vi "sub_CMC Match.vi"(8 "error in (no error)":errorcluster caption="에러 입력(에러 없음)", 10 "DATA IN":string[][](array[string]), 11 "CMC IN":string[][](array[string])) -> (0 "error out":errorcluster caption="에러 출력", 2 "에러?":bool, 3 "CMC Out":string[][](array[string]))   [LabVIEW 2020]
panel:
  out "배열":bool[](array[boolean])
  # "0, DSEQ\n1, CLSMAN\n2, CLSMAN_EXT\n3, FUNC\n4, FUNC_EXT\n5, FUNC_CON\n6, C1_LOW\n7, C1_LUNIT\n8, C1_LCON\n9, C1_HIGH\n10, C1_HUNIT\n11, C1_HCON\n12, RANGE_LOW\n13, RANGE_LUNIT\n14, RANGE_LDIV\n15, RANGE_HIGH\n16, RANGE_HUNIT\n17, RANGE_HDIV\n18, CMC1_VAL\n19, CMC2_VAL\n20, CMC_UNIT"
  # "0, CLSMAN_EXT\n1, FUNC\n2, FUNC_EXT\n3, FUNC_CON\n4, C1_VAL\n5, C1_UNIT\n6, RANGE_VAL\n7, RANGE_UNIT"
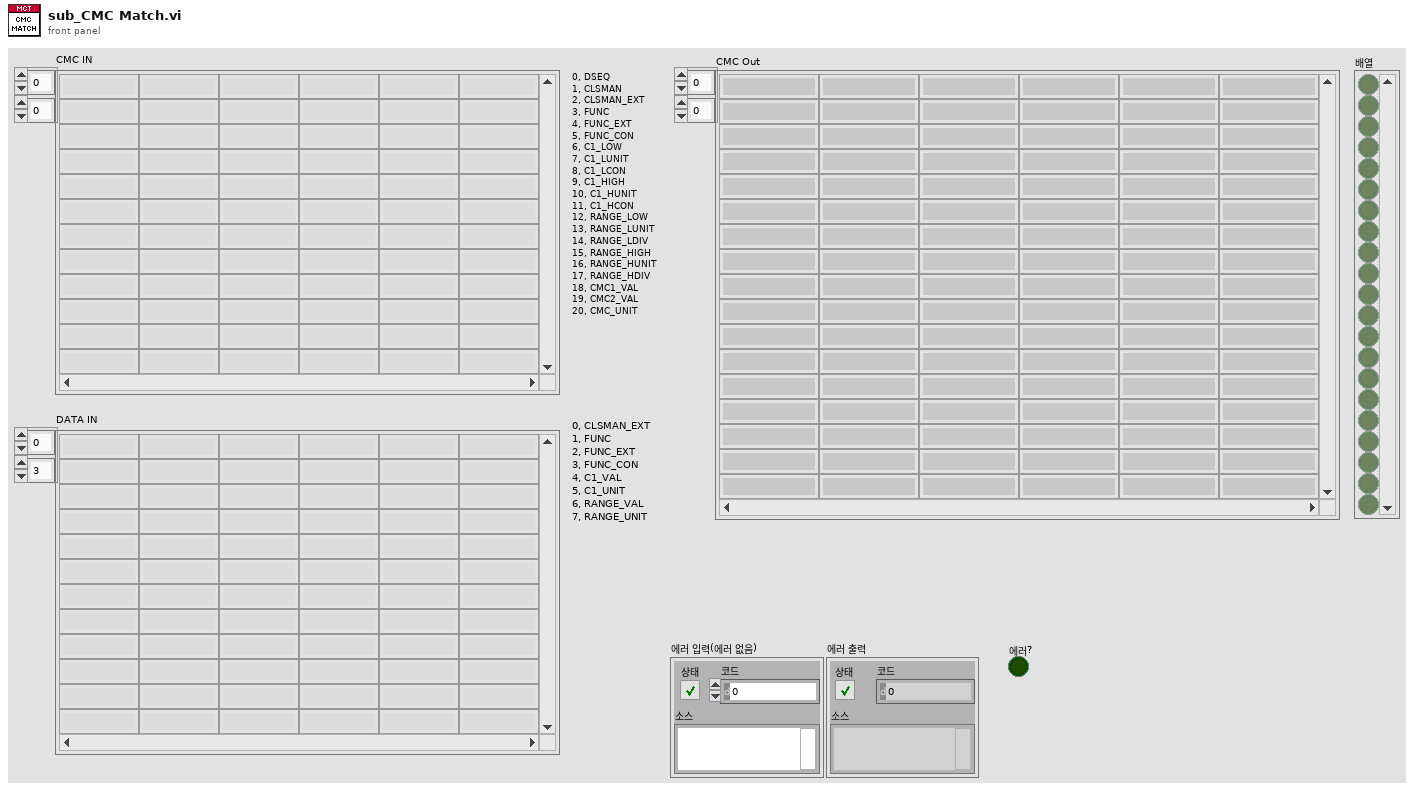
[diagram p1: front panel]
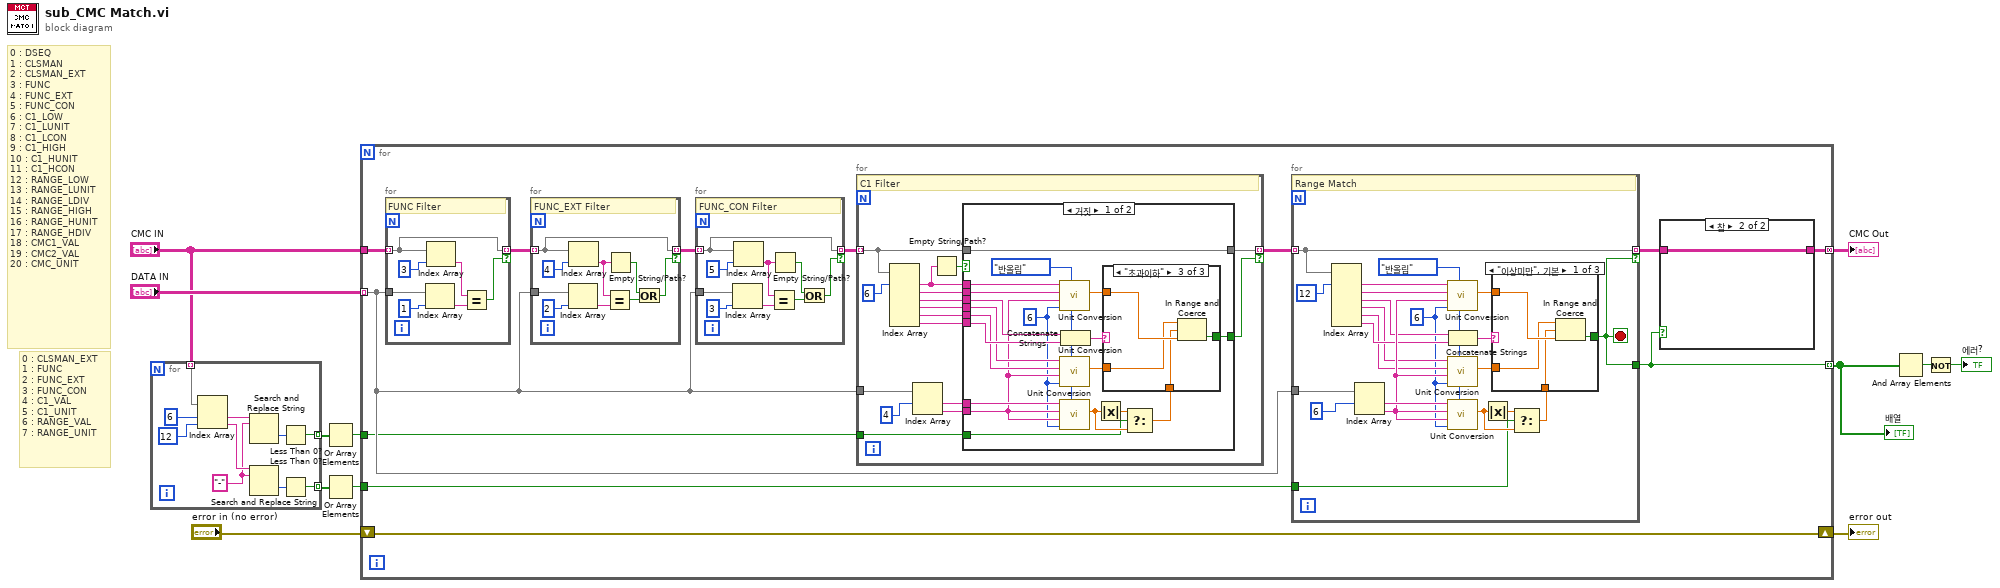
[diagram p0: block diagram]
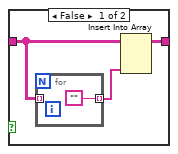
[diagram p2: hidden frame]
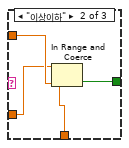
[diagram p3: hidden frame]
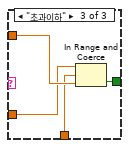
[diagram p4: hidden frame]
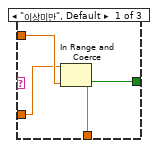
[diagram p5: hidden frame]
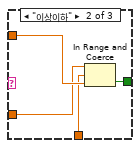
[diagram p6: hidden frame]
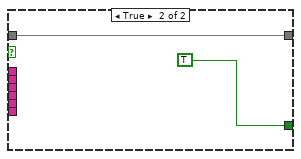
[diagram p7: hidden frame]
diagram:
  # "0 : CLSMAN_EXT\n1 : FUNC\n2 : FUNC_EXT\n3 : FUNC_CON\n4 : C1_VAL\n5 : C1_UNIT\n6 : RANGE_VAL\n7 : RANGE_UNIT"
  # "0 : DSEQ\n1 : CLSMAN\n2 : CLSMAN_EXT\n3 : FUNC\n4 : FUNC_EXT\n5 : FUNC_CON\n6 : C1_LOW\n7 : C1_LUNIT\n8 : C1_LCON\n9 : C1_HIGH\n10 : C1_HUNIT\n11 : C1_HCON\n12 : RANGE_LOW\n13 : RANGE_LUNIT\n14 : RANGE_LDIV\n15 : RANGE_HIGH\n16 : RANGE_HUNIT\n17 : RANGE_HDIV\n18 : CMC1_VAL\n19 : CMC2_VAL\n20 : CMC_UNIT"
  n1 = for {
    tunnel: "CMC IN" -> [w22] mode=indexing
    tunnel: [w18] -> w6 mode=indexing
    tunnel: [w13] -> w5 mode=indexing
    w15 = "-" ("검색 문자열")
    n2 = Index Array(array=w22, index #1=6 ("비활성화된 인덱스 (열)"), index #2=12 ("비활성화된 인덱스 (열)")) -> (element #1=w16:string, element #2=w20:string)
    n3 = Search and Replace String(input string=w16, search string=w15) -> (offset past replacement=w14:i32)  [unwired: 6 in, 3 out]
    n4 = Search and Replace String(input string=w20, search string=w15) -> (offset past replacement=w19:i32)  [unwired: 6 in, 3 out]
    n5 = Less Than 0?(x=w14) -> (x < 0?=w13:bool)
    n6 = Less Than 0?(x=w19) -> (x < 0?=w18:bool)
  }
  n7 = Or Array Elements(Boolean array=w5) -> (logical OR=w2:bool)
  n8 = Or Array Elements(Boolean array=w6) -> (logical OR=w1:bool)
  n9 = for {
    tunnel: "DATA IN" -> [w25] mode=indexing
    tunnel: "CMC IN" -> [w34]
    tunnel: [w28] -> w12 mode=concatenating
    shift-right: [w31] -> w10
    shift-left: "error in (no error)" -> [w31]
    tunnel: [w30] -> w9 mode=indexing
    tunnel: w2 -> [w24]
    tunnel: w1 -> [w23]
    n10 = for {
      tunnel: w34 -> [w146] mode=indexing
      tunnel: w25 -> [w147]
      tunnel: [w146] -> w33 mode=indexing if=w145
      # "FUNC Filter"
      n11 = Index Array(array=w147, index=1 ("인덱스")) -> (element=w143:string)
      n12 = Index Array(array=w146, index=3 ("인덱스")) -> (element=w144:string)
      n13 = Equal?(x=w144, y=w143) -> (x = y?=w145:bool)
    }
    n14 = for {
      tunnel: w33 -> [w139] mode=indexing
      tunnel: w25 -> [w140]
      tunnel: [w139] -> w27 mode=indexing if=w132
      # "FUNC_EXT Filter"
      n15 = Index Array(array=w140, index=2 ("인덱스")) -> (element=w137:string)
      n16 = Index Array(array=w139, index=4 ("인덱스")) -> (element=w135:string)
      n17 = Equal?(x=w135, y=w137) -> (x = y?=w134:bool)
      n18 = Empty String/Path?(string/path=w135) -> (empty?=w133:bool)
      n19 = Or(x=w133, y=w134) -> (x .or. y?=w132:bool)
    }
    n20 = for {
      tunnel: w27 -> [w42] mode=indexing
      tunnel: w25 -> [w43]
      tunnel: [w42] -> w26 mode=indexing if=w35
      # "FUNC_CON Filter"
      n21 = Index Array(array=w43, index=3 ("인덱스")) -> (element=w40:string)
      n22 = Index Array(array=w42, index=5 ("인덱스")) -> (element=w38:string)
      n23 = Equal?(x=w38, y=w40) -> (x = y?=w37:bool)
      n24 = Empty String/Path?(string/path=w38) -> (empty?=w36:bool)
      n25 = Or(x=w36, y=w37) -> (x .or. y?=w35:bool)
    }
    n26 = for {
      tunnel: w26 -> [w95] mode=indexing
      tunnel: w25 -> [w98]
      tunnel: [w94] -> w32 mode=indexing if=w88
      tunnel: w24 -> [w83]
      # "C1 Filter"
      n27 = Index Array(array=w95, index #1=6 ("인덱스")) -> (element #1=w92:string, element #2=w91:string, element #3=w89:string, element #4=w86:string, element #5=w85:string, element #6=w87:string)  [unwired: 5 in]
      n28 = Index Array(array=w98, index #1=4 ("인덱스")) -> (element #1=w93:string, element #2=w90:string)  [unwired: 1 in]
      n29 = Empty String/Path?(string/path=w92) -> (empty?=w96:bool)
      n30 = case shown="거짓" w96 {
        tunnel: w95 -> [w104 w131]
        tunnel: [w104 w131] -> w94
        tunnel: w93 -> [w108 _]
        tunnel: w92 -> [w117 _]
        tunnel: w91 -> [w116 _]
        tunnel: w90 -> [w107 _]
        tunnel: w89 -> [w115 _]
        tunnel: [w106 TRUE] -> w88
        tunnel: w87 -> [w114 _]
        tunnel: w86 -> [w111 _]
        tunnel: w85 -> [w110 _]
        tunnel: w83 -> [w99 _]
        frame False {
          w105 = 6 ("소수점 자리수")
          w103 = enum16{"없음", "반올림", "올림", "내림"}."반올림" ("반올림 옵션")
          n31 = call "Unit Conversion.vi"("반올림 옵션"=w103, "소수점 자리수"=w105, "환산단위"=w107, "입력단위"=w116, "입력값"=w117) -> ("환산값 (DBL)"=w112:dbl)  [unwired: 1 in, 5 out]
          n32 = call "Unit Conversion.vi"("반올림 옵션"=w103, "소수점 자리수"=w105, "환산단위"=w107, "입력단위"=w110, "입력값"=w111) -> ("환산값 (DBL)"=w109:dbl)  [unwired: 1 in, 5 out]
          n33 = call "Unit Conversion.vi"("반올림 옵션"=w103, "소수점 자리수"=w105, "환산단위"=w107, "입력단위"=w107, "입력값"=w108) -> ("환산값 (DBL)"=w101:dbl)  [unwired: 1 in, 5 out]
          n34 = Concatenate Strings(w115, w114) -> (w113:string)
          n35 = Absolute Value(x=w101) -> (abs(x)=w102:dbl)
          n36 = Select(t=w102, s=w99, f=w101) -> (s? t:f=w100:dbl)
          n37 = case shown="\"초과이하\"" w113 {
            tunnel: w112 -> [w121 w124 w129]
            tunnel: w109 -> [w120 w123 w127]
            tunnel: w100 -> [w119 w122 w128]
            tunnel: [w118 w125 w126] -> w106
            frame "이상미만", Default {
              n38 = In Range and Coerce(upper limit=w120, x=w119, lower limit=w121) -> (In Range?=w118:bool)  [unwired: 1 out]
            }
            frame "이상이하" {
              n39 = In Range and Coerce(upper limit=w123, x=w122, lower limit=w124) -> (In Range?=w125:bool)  [unwired: 1 out]
            }
            frame "초과이하" {
              n40 = In Range and Coerce(upper limit=w127, x=w128, lower limit=w129) -> (In Range?=w126:bool)  [unwired: 1 out]
            }
          }
        }
        frame True {
        }
      }
    }
    n41 = for {
      tunnel: w32 -> [w54] mode=indexing
      tunnel: w25 -> [w70]
      tunnel: [w54] -> w29 mode=indexing if=w53
      tunnel: [w53] -> w30
      tunnel: w23 -> [w49]
      stop <- w53 stop-if-true
      w55 = 6 ("소수점 자리수")
      w56 = enum16{"없음", "반올림", "올림", "내림"}."반올림" ("반올림 옵션")
      # "Range Match"
      n42 = Index Array(array=w54, index #1=12 ("인덱스")) -> (element #1=w67:string, element #2=w66:string, element #3=w64:string, element #4=w62:string, element #5=w61:string, element #6=w63:string)  [unwired: 5 in]
      n43 = Index Array(array=w70, index #1=6 ("인덱스")) -> (element #1=w68:string, element #2=w65:string)  [unwired: 1 in]
      n44 = call "Unit Conversion.vi"("반올림 옵션"=w56, "소수점 자리수"=w55, "환산단위"=w65, "입력단위"=w66, "입력값"=w67) -> ("환산값 (DBL)"=w58:dbl)  [unwired: 1 in, 5 out]
      n45 = call "Unit Conversion.vi"("반올림 옵션"=w56, "소수점 자리수"=w55, "환산단위"=w65, "입력단위"=w61, "입력값"=w62) -> ("환산값 (DBL)"=w57:dbl)  [unwired: 1 in, 5 out]
      n46 = call "Unit Conversion.vi"("반올림 옵션"=w56, "소수점 자리수"=w55, "환산단위"=w65, "입력단위"=w65, "입력값"=w68) -> ("환산값 (DBL)"=w51:dbl)  [unwired: 1 in, 5 out]
      n47 = Concatenate Strings(w64, w63) -> (w59:string)
      n48 = Absolute Value(x=w51) -> (abs(x)=w52:dbl)
      n49 = Select(t=w52, s=w49, f=w51) -> (s? t:f=w50:dbl)
      n50 = case shown="\"이상미만\", 기본" w59 {
        tunnel: w58 -> [w74 w77 w82]
        tunnel: w57 -> [w73 w76 w80]
        tunnel: w50 -> [w72 w75 w81]
        tunnel: [w71 w78 w79] -> w53
        frame "이상미만", Default {
          n51 = In Range and Coerce(upper limit=w73, x=w72, lower limit=w74) -> (In Range?=w71:bool)  [unwired: 1 out]
        }
        frame "이상이하" {
          n52 = In Range and Coerce(upper limit=w76, x=w75, lower limit=w77) -> (In Range?=w78:bool)  [unwired: 1 out]
        }
        frame "초과이하" {
          n53 = In Range and Coerce(upper limit=w80, x=w81, lower limit=w82) -> (In Range?=w79:bool)  [unwired: 1 out]
        }
      }
    }
    n54 = case shown="참" w30 {
      tunnel: w29 -> [w46 w48]
      tunnel: [w45 w48] -> w28
      frame False {
        n55 = for {
          tunnel: [""] -> w44 mode=indexing
          tunnel: w46 -> [_] mode=indexing
        }
        n56 = Insert Into Array(array=w46, new element=w44) -> (w45:string[][])  [unwired: 2 in]
      }
      frame True {
      }
    }
  }
  "error out" <- w10
  "CMC Out" <- w12
  "배열" <- w9
  n57 = And Array Elements(Boolean array=w9) -> (logical AND=w8:bool)
  n58 = Not(x=w8) -> (.not. x?=→"에러?":bool)
